vi "Piece of Bricks_Init.vi"(8 "error in (no error)":errorcluster) -> (0 "error out":errorcluster, 3 "object out":refnum<class "Piece of Bricks.lvclass">)   [LabVIEW 2017, in "Piece of Bricks.lvclass"]
uses:
  Piece of Bricks.lvclass
  Piece of Bricks.lvclass/Piece of Bricks.ctl
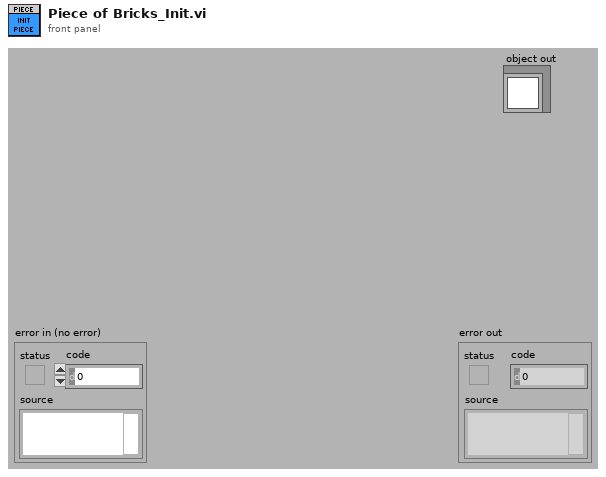
[diagram p1: front panel]
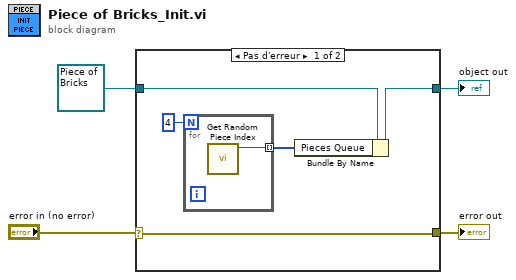
[diagram p0: block diagram]
diagram:
  n1 = case shown="Pas d'erreur" "error in (no error)" {
    selector: "error in (no error)" -> [w8 w11]
    tunnel: [w9 w12] -> w4
    tunnel: refnum<class "Piece of Bricks.lvclass"> refnum ("object in") -> [w7 w12]
    tunnel: [w8 w11] -> w1
    frame No Error {
      n2 = for {
        N: 4 -> [_]
        tunnel: [w10] -> w6 mode=indexing
        n3 = call "Get Random Piece Index.vi"() -> ("Piece index"=w10:u16)  [unwired: 10 in, 1 out]
      }
      n4 = Bundle By Name(cluster=w7, "Pieces Queue"=w6) -> (w9:refnum<class "Piece of Bricks.lvclass">)
    }
    frame Error {
    }
  }
  "object out" <- w4
  "error out" <- w1
